vi "Rinocloud_explorer.vi"() -> ()   [LabVIEW 2013, in "Rinocloud Library.lvlib"]
uses:
  Rinocloud Library.lvlib
  Rinocloud_global_variable.vi
panel:
  out "Last action:":string
  out "error out":errorcluster
  in  "Active item:":string="<folder> home (id=)"
  in  "delete":bool
  in  "refresh list":bool
  in  "Tab Control":T1(tab)=enum."HTTP"
  in  "Cluster 2":T2={"Attribute"="", "Value"="", "Data type"=5} {"Data type" items=["Numeric", "String", "1D array of strings", "1D array of doubles", "Data JSON string", "<null>"]}
  in  "Cluster 1":T2={"Attribute"="", "Value"="", "Data type"=5} {"Data type" items=["Numeric", "String", "1D array of strings", "1D array of doubles", "Data JSON string", "<null>"]}
  in  "name":string
  in  "tags":string
  in  "notes":string
  in  "new folder":bool
  in  "upload file":bool
  in  "Name:":string
  in  "Tags:":string
  in  "Notes:":string
  in  "get metadata":bool
  in  "metadata tree":string(tree) caption="Metadata"
  in  "update metadata":bool
  in  "Move":bool
  in  "Destination:":string
  in  "Source:":string
  in  "set source":bool
  in  "set destination":bool
  out "body":string
  out "headers":string
  in  "ancestor tree":string(tree)="home" caption="Active path"
  in  "stop":bool
  in  "active child tree":string(tree) caption="File & folder list of the active folder"
  # "Double-click an item to activate"
  # "Custom metadata:"
  # "(tag1,tag2,tag3,...)"
  # "Click the fields to edit"
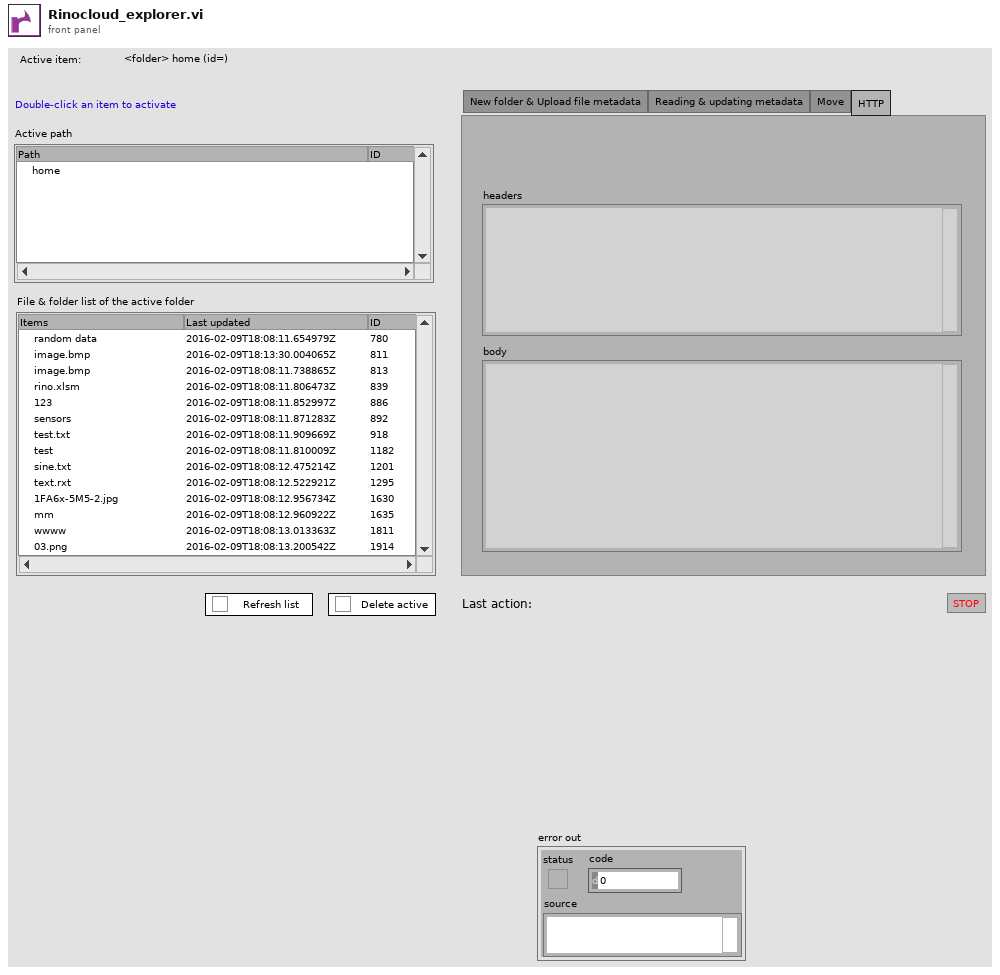
[diagram p1: front panel]
types:
  T1 = enum32{"New folder & Upload file metadata", "Reading & updating metadata", "Move", "HTTP"}
  T2 = cluster{"Attribute":string, "Value":string, "Data type":u16}
  T3 = cluster{"Active items":cluster{"Active file ID":string, "Active dir ID":string, "Active object ID":string, "Recent ID":string, "Active item:":string, "Source item":string, "Destination item":string, "Source ID":string, "Destination ID":string}, "Trees":cluster{"Ancestors":refnum<vi>, "Children":refnum<vi>, "Metadata":refnum<vi>}, "New metadata":cluster{"Name":string, "Tags":string, "Notes":string, "Custom metadata":cluster{"Attribute":string, "Value":string, "Data type":u16}[]}, "Communication":cluster{"HTTP headers":string, "HTTP body":string, "Project name":string, "User":string}, "Controls":cluster{"Move refnum":refnum<vi>}, "Status messages":cluster{"error ":errorcluster, "status":string}, "Update metadata":cluster{"Name":string, "Tags":string, "Notes":string}}
  T4 = enum16{"Boot", "Initialize", "Wait for event", "Refresh", "Metadata to tree", "Stop"}
  T5 = cluster{"Active file ID":string, "Active dir ID":string, "Active object ID":string, "Recent ID":string, "Active item:":string, "Source item":string, "Destination item":string, "Source ID":string, "Destination ID":string}
  T6 = enum8{"Enabled", "Disabled", "Disabled and Grayed Out"}
  T7 = cluster{"HTTP headers":string, "HTTP body":string, "Project name":string, "User":string}
  T8 = cluster{"Name":string, "Tags":string, "Notes":string, "Custom metadata":cluster{"Attribute":string, "Value":string, "Data type":u16}[]}
  T9 = enum16{"Boot", "Initialize", "Wait for event", "Refresh", "Stop"}
  T10 = cluster{"Store locally":bool, "ancestor array":cluster{"id":string, "name":string, "created_on":string, "updated_on":string, "tags":string, "notes":string, "record type":string, "metadata (JSON)":string}[], "Store metadata":bool}
  T11 = cluster{"Attribute":string, "Value":string, "Data type":enum16{"Numeric", "String", "1D array of strings", "1D array of doubles", "Data JSON string", "<null>"}}[]
  T12 = cluster{"headers":string, "body":string, "ID":string, "Saved":bool}
  T13 = cluster{"Attribute":string, "Value":string, "Data type":u16}[]
  T14 = cluster{"id":string, "name":string, "created_on":string, "updated_on":string, "tags":string, "notes":string, "record type":string, "metadata (JSON)":string}[]
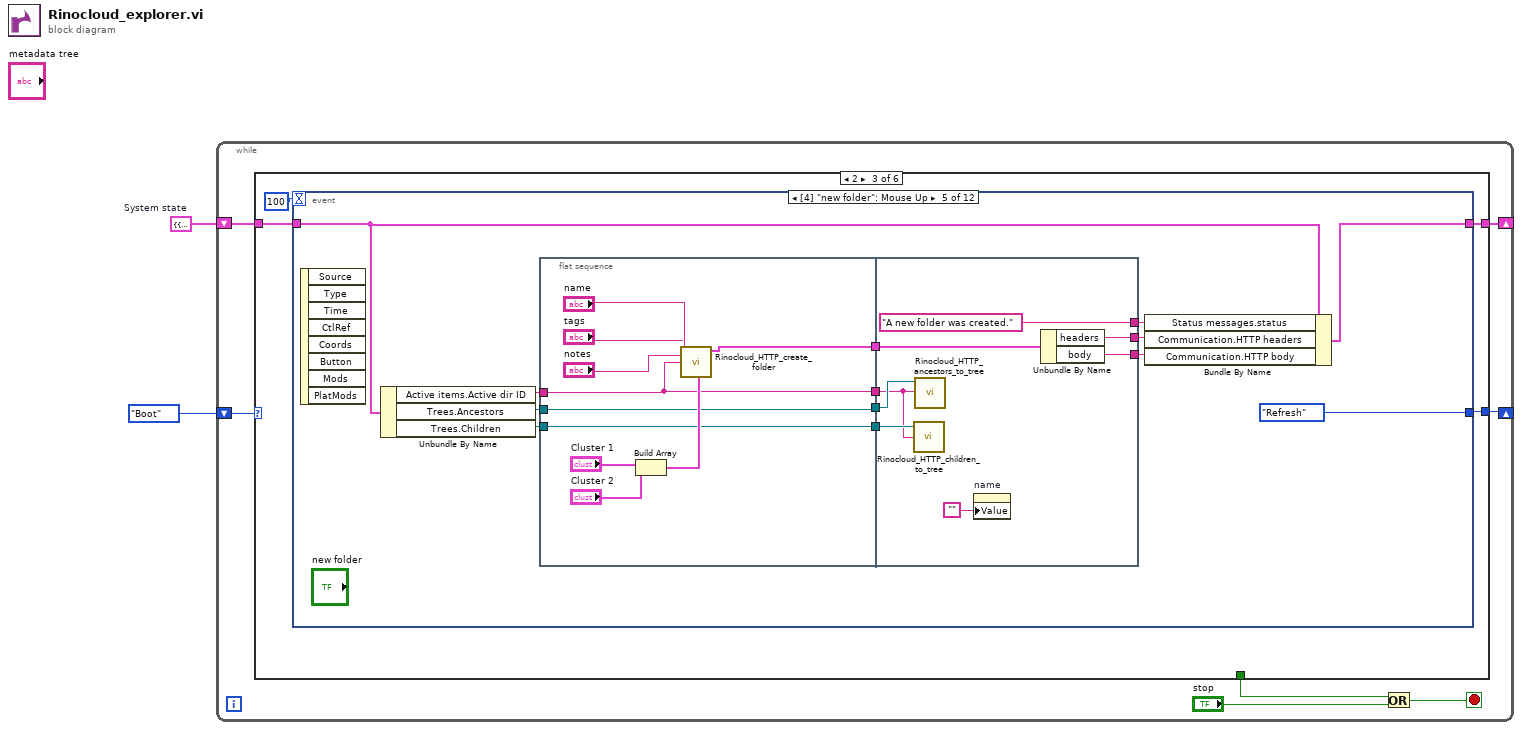
[diagram p0: block diagram]
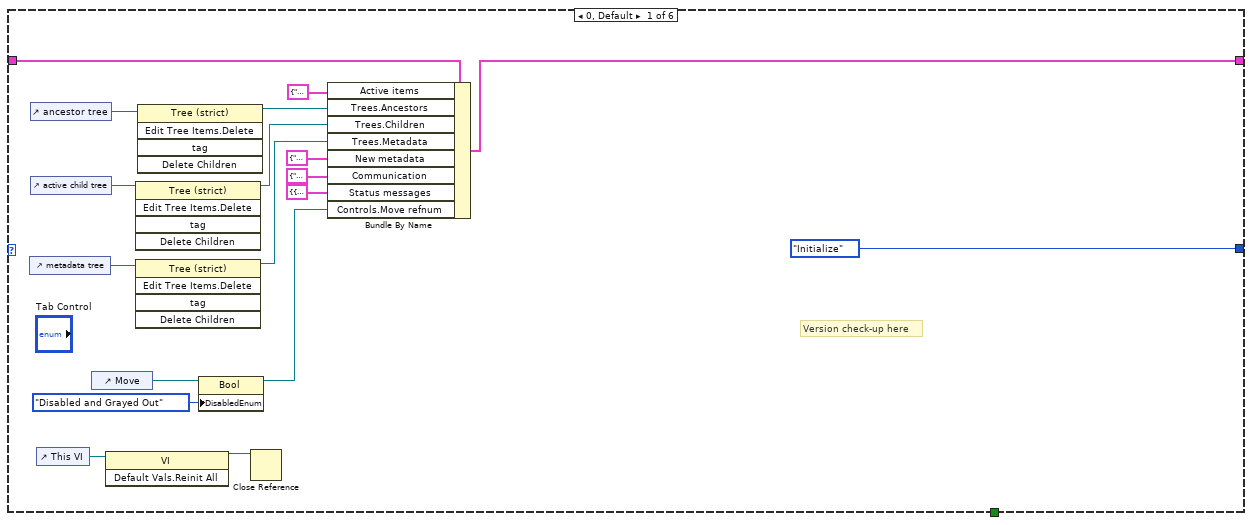
[diagram p2: hidden frame]
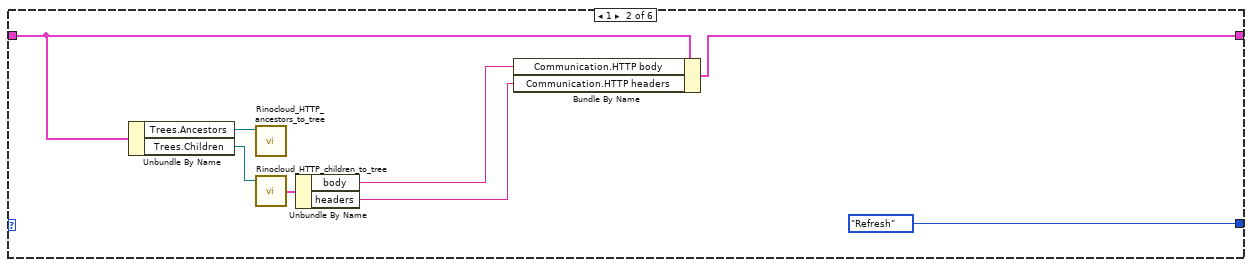
[diagram p3: hidden frame]
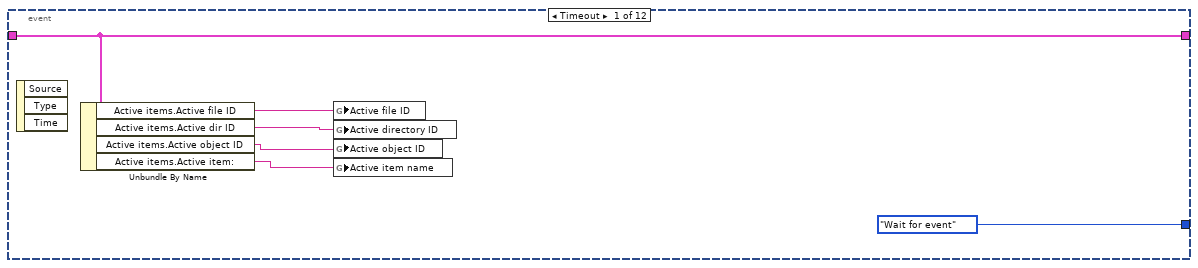
[diagram p4: hidden frame]
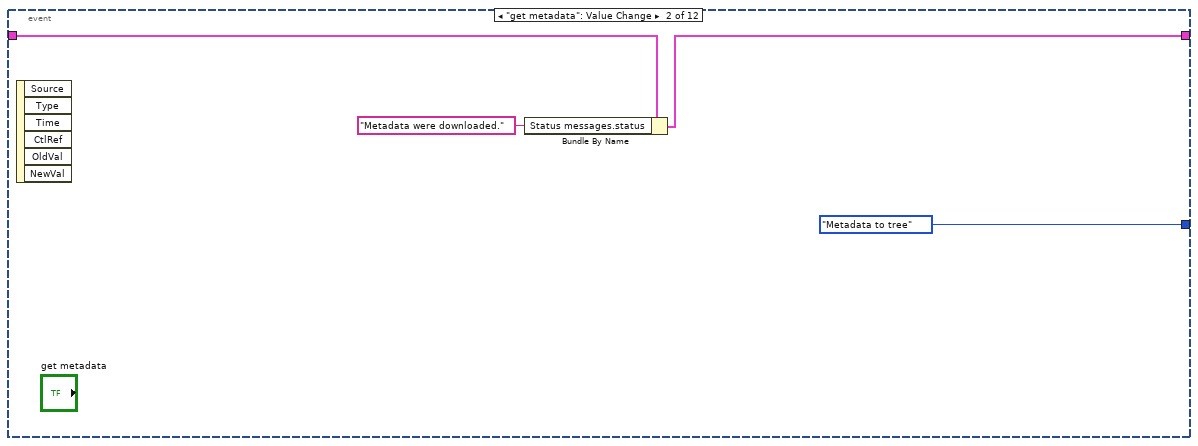
[diagram p5: hidden frame]
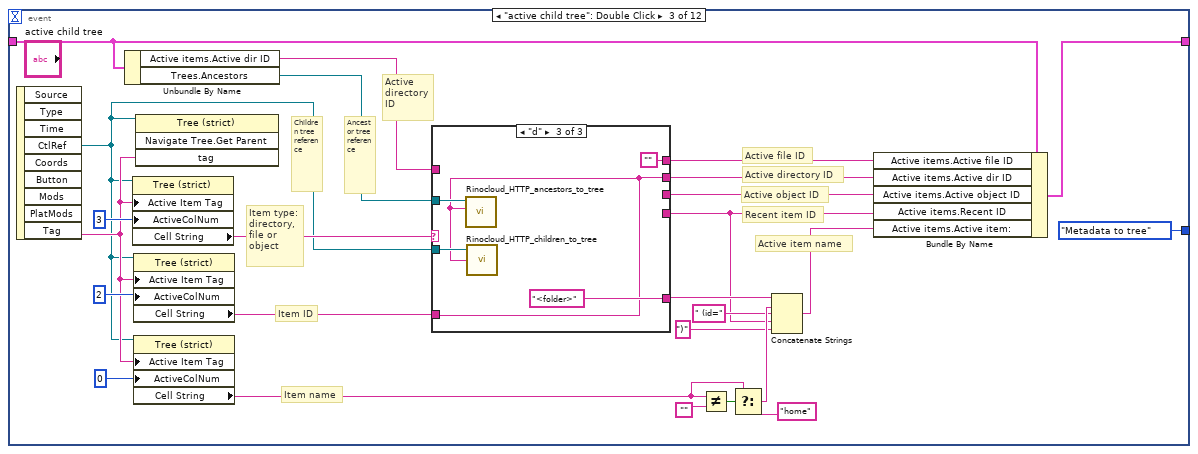
[diagram p6: hidden frame]
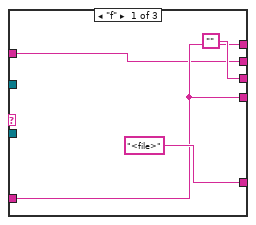
[diagram p7: hidden frame]
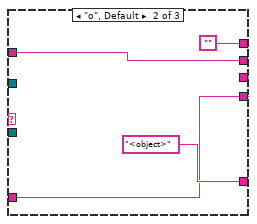
[diagram p8: hidden frame]
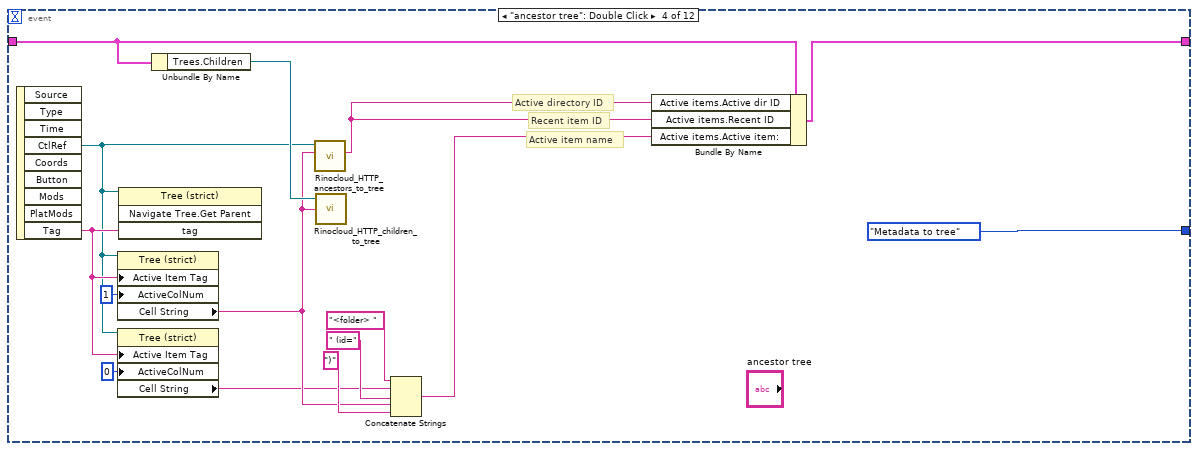
[diagram p9: hidden frame]
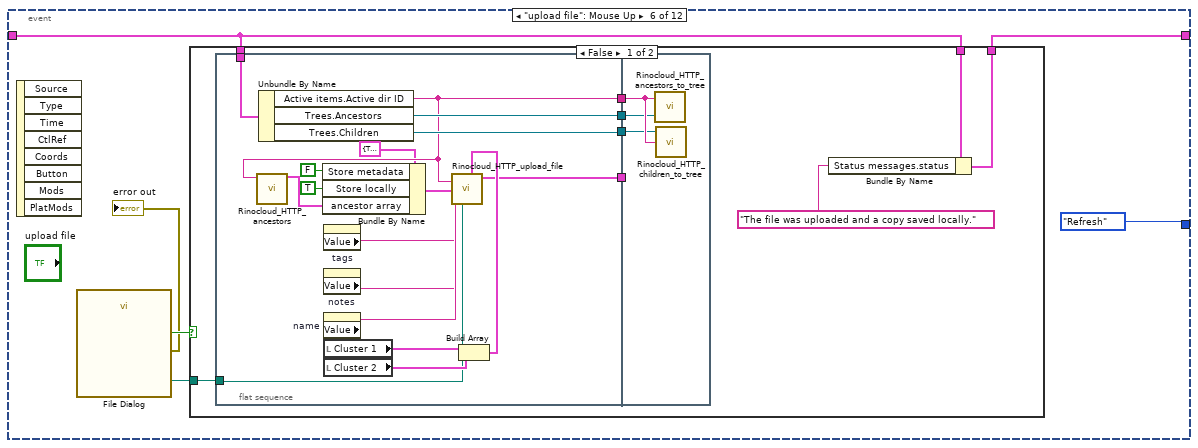
[diagram p10: hidden frame]
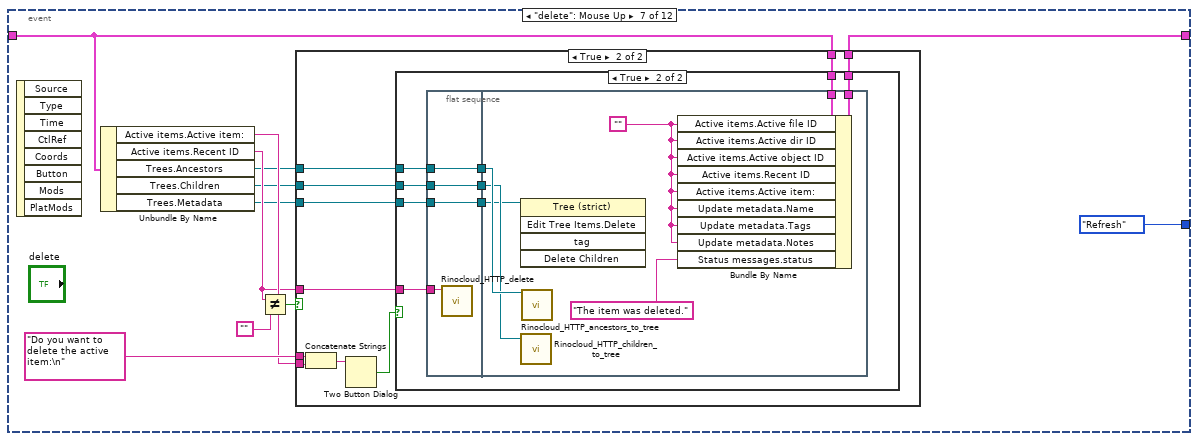
[diagram p12: hidden frame]
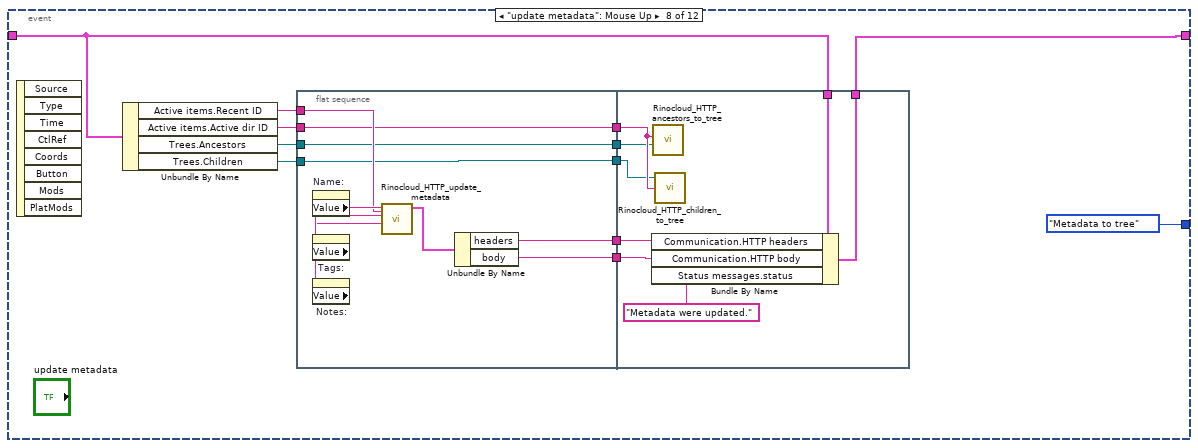
[diagram p15: hidden frame]
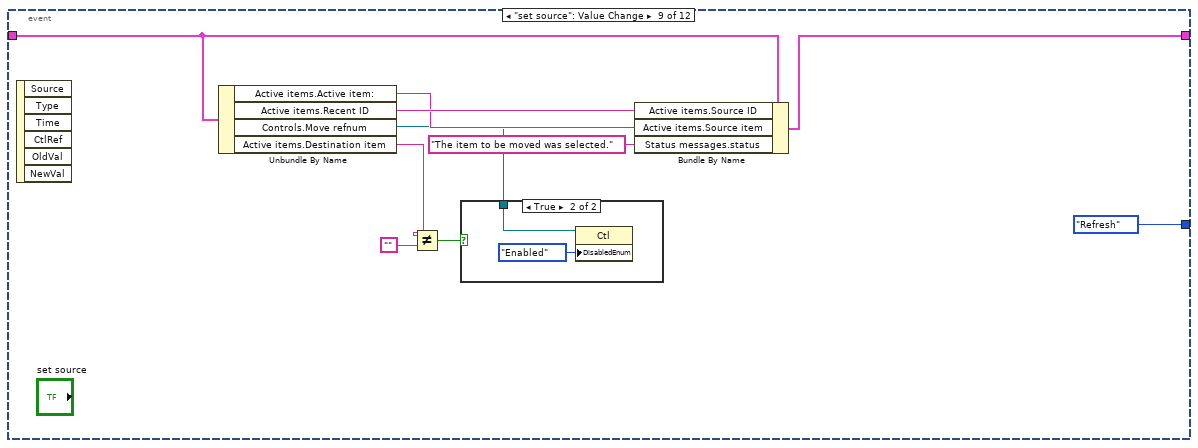
[diagram p16: hidden frame]
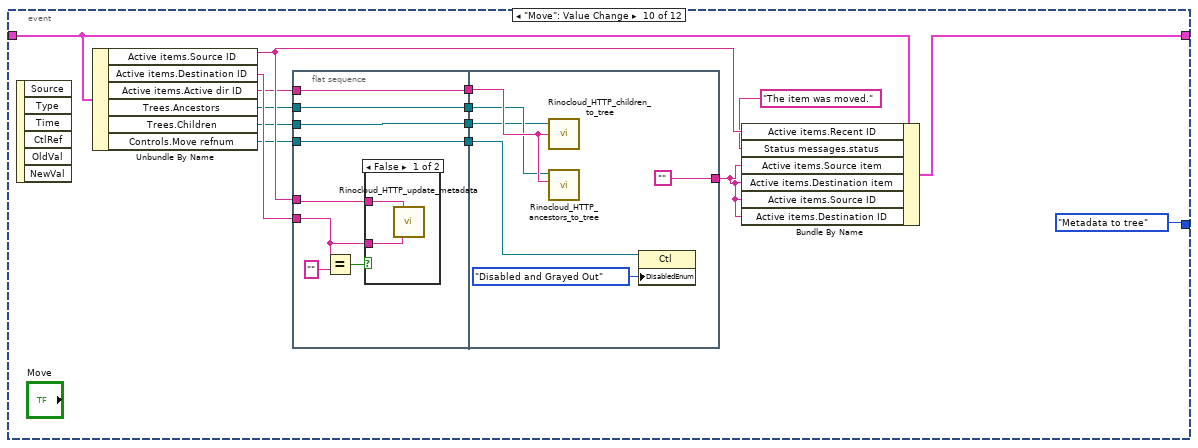
[diagram p18: hidden frame]
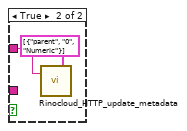
[diagram p19: hidden frame]
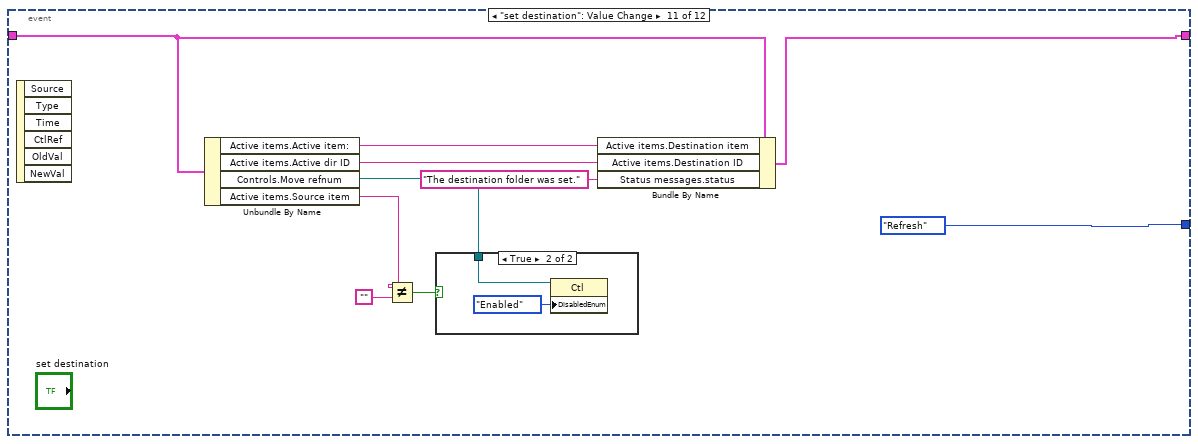
[diagram p20: hidden frame]
diagram:
  w2 = T3 {"Active items"={"Active file ID"="", "Active dir ID"="", "Active object ID"="", "Recent ID"="", "Active item:"="<folder> home (id=)", "Source item"="", "Destination item"="", "Source ID"="", "Destination ID"=""}, "Trees"={"Ancestors"=refnum, "Children"=refnum, "Metadata"=refnum}, "New metadata"={"Name"="", "Tags"="", "Notes"="", "Custom metadata"=[]}, "Communication"={"HTTP headers"="", "HTTP body"="", "Project name"="", "User"=""}, "Controls"={"Move refnum"=refnum}, "Status messages"={"error "={"status"=FALSE, "code"=0, "source"=""}, "status"=""}, "Update metadata"={"Name"="", "Tags"="", "Notes"=""}}  # System state
  n1 = while {
    shift-right: [w3] -> _
    shift-left: T4."Boot" -> [w9]
    shift-right: [w4] -> _
    shift-left: w2 -> [w5]
    stop <- w8 stop-if-true
    n2 = case shown="2" w9 {
      tunnel: [T4."Initialize" T9."Refresh" w38 T9."Wait for event" T4."Stop" T4."Refresh"] -> w3
      tunnel: [_ _ _ _ TRUE _] -> w6
      tunnel: w5 -> [w27 w32 w37 w312 w316 w324]
      tunnel: [w18 w29 w36 w312 w316 w323] -> w4
      frame 0, Default {
        # "Version check-up here"
        n3 = control-ref of="metadata tree"() -> (w22:refnum<vi>)
        n4 = control-ref of="ancestor tree"() -> (w26:refnum<vi>)
        n5 = control-ref of="active child tree"() -> (w24:refnum<vi>)
        n6 = control-ref of="This VI"() -> (w13:refnum<vi>)
        n7 = control-ref of="Move"() -> (w17:refnum<vi>)
        n8 = invoke class="VI" method="Default Vals.Reinit All"(reference=w13) -> (reference out=w12:refnum<vi>)  [unwired: 2 in, 2 out]
        n9 = invoke class="Tree (strict)" method="Edit Tree Items.Delete"(reference=w24) -> (reference out=w23:refnum<vi>)  [unwired: 4 in, 4 out]
        n10 = invoke class="Tree (strict)" method="Edit Tree Items.Delete"(reference=w22) -> (reference out=w11:refnum<vi>)  [unwired: 4 in, 4 out]
        n11 = invoke class="Tree (strict)" method="Edit Tree Items.Delete"(reference=w26) -> (reference out=w25:refnum<vi>)  [unwired: 4 in, 4 out]
        n12 = property class="Bool"(reference=w17, "DisabledEnum"=T6."Disabled and Grayed Out" ("Disabled")) -> (reference out=w15:refnum<vi>)  [unwired: 1 in, 1 out]
        n13 = Close Reference(reference=w12) -> ()  [unwired: 1 in, 1 out]
        n14 = Bundle By Name(cluster=w27, "Active items"=T5 {"Active file ID"="", "Active dir ID"="", "Active object ID"="", "Recent ID"="", "Active item:"="<folder> home (id=)", "Source item"="", "Destination item"="", "Source ID"="", "Destination ID"=""}, "Trees.Ancestors"=w25, "Trees.Children"=w23, "Trees.Metadata"=w11, "New metadata"=T8 {"Name"="", "Tags"="", "Notes"="", "Custom metadata"=[]} ("Metadata"), "Communication"=T7 {"HTTP headers"="", "HTTP body"="", "Project name"="", "User"=""}, "Status messages"=cluster{"error ":errorcluster, "status":string} {"error "={"status"=FALSE, "code"=0, "source"=""}, "status"=""}, "Controls.Move refnum"=w15) -> (w18:T3)
      }
      frame 1 {
        n15 = Unbundle By Name(w32) -> ("Trees.Ancestors"=w33:refnum<vi>, "Trees.Children"=w34:refnum<vi>)
        n16 = call "Rinocloud_HTTP_ancestors_to_tree.vi"("Tree Ref in"=w33) -> ()  [unwired: 3 in, 4 out]
        n17 = call "Rinocloud_HTTP_children_to_tree.vi"("Tree Ref in"=w34) -> ("Status"=w35:T12)  [unwired: 2 in, 2 out]
        n18 = Unbundle By Name(w35) -> ("body"=w31:string, "headers"=w30:string)
        n19 = Bundle By Name(cluster=w32, "Communication.HTTP body"=w31, "Communication.HTTP headers"=w30) -> (w29:T3)
      }
      frame 2 {
        n20 = event shown="[4] \"new folder\": Mouse Up" {
          selector: _ -> [_ _ _ _ _ _ _ _ _ _ _ _]
          dyn-events: _ -> [_ _ _ _ _ _ _ _ _ _ _ _]
          timeout: 100 -> [_ _ _ _ _ _ _ _ _ _ _ _]
          tunnel: [T9."Wait for event" T4."Metadata to tree" T4."Metadata to tree" T4."Metadata to tree" T4."Refresh" T4."Refresh" T4."Refresh" T4."Metadata to tree" T4."Refresh" T4."Metadata to tree" T4."Refresh" T4."Initialize"] -> w38
          tunnel: w37 -> [w40 w47 w62 w97 w108 w136 w172 w216 w252 w267 w292 w301]
          tunnel: [w40 w46 w59 w95 w107 w135 w170 w213 w244 w258 w288 w300] -> w36
          event Timeout {
            n21 = event-data() -> ()  [unwired: 1 in, 3 out]
            n22 = Unbundle By Name(w40) -> ("Active items.Active file ID"=w45:string, "Active items.Active dir ID"=w44:string, "Active items.Active object ID"=w43:string, "Active items.Active item:"=w41:string)
            n23 = global write "Rinocloud_global_variable.vi" "Active file ID"(w45) -> ()
            n24 = global write "Rinocloud_global_variable.vi" "Active directory ID"(w44) -> ()
            n25 = global write "Rinocloud_global_variable.vi" "Active object ID"(w43) -> ()
            n26 = global write "Rinocloud_global_variable.vi" "Active item name"(w41) -> ()
          }
          event "get metadata": Value Change {
            n27 = event-data() -> ()  [unwired: 1 in, 6 out]
            n28 = Bundle By Name(cluster=w47, "Status messages.status"="Metadata were downloaded.") -> (w46:T3)
          }
          event "active child tree": Double Click {
            # "Active \ndirectory\nID"
            # "Ancestor tree \nreference"
            # "Children tree \nreference"
            # "Item name"
            # "Item type:\ndirectory,\nfile or\nobject"
            # "Item ID"
            # "Active item name"
            # "Recent item ID"
            # "Active object ID"
            # "Active directory ID"
            # "Active file ID"
            n29 = event-data() -> ("CtlRef"=w50:refnum<vi>, "Tag"=w55:string)  [unwired: 1 in, 7 out]
            n30 = Unbundle By Name(w62) -> ("Active items.Active dir ID"=w60:string, "Trees.Ancestors"=w61:refnum<vi>)
            n31 = property on="Property Node" class="Tree (strict)"(reference=w50, "Active Item Tag"=w55, "ActiveColNum"=3 ("Active Cell:Active Column Number")) -> ("Cell String"=w54:string)  [unwired: 1 in, 2 out]
            n32 = property on="Property Node" class="Tree (strict)"(reference=w50, "Active Item Tag"=w55, "ActiveColNum"=2 ("Active Cell:Active Column Number")) -> ("Cell String"=w53:string)  [unwired: 1 in, 2 out]
            n33 = property on="Property Node" class="Tree (strict)"(reference=w50, "Active Item Tag"=w55, "ActiveColNum"=0 ("Active Cell:Active Column Number")) -> ("Cell String"=w52:string)  [unwired: 1 in, 2 out]
            n34 = invoke on="Invoke Node" class="Tree (strict)" method="Navigate Tree.Get Parent"(reference=w50, "tag"=w55) -> ()  [unwired: 2 in, 4 out]
            n35 = case shown="\"d\"" w54 {
              tunnel: w53 -> [w76 w81 w83]
              tunnel: ["<file>" ("f") "<object>" ("f") "<folder>" ("f")] -> w70
              tunnel: [w76 w81 w83] -> w64
              tunnel: ["" w81 w86] -> w65
              tunnel: [w76 "" w86] -> w51
              tunnel: [w75 w79 w83] -> w63
              tunnel: w61 -> [_ _ w85]
              tunnel: w50 -> [_ _ w84]
              tunnel: w60 -> [w75 w79 _]
              frame "f" {
              }
              frame "o", Default {
              }
              frame "d" {
                w86 = ""
                n36 = call "Rinocloud_HTTP_ancestors_to_tree.vi"("id"=w83, "Tree Ref in"=w85) -> ()  [unwired: 2 in, 4 out]
                n37 = call "Rinocloud_HTTP_children_to_tree.vi"("id"=w83, "Tree Ref in"=w84) -> ()  [unwired: 1 in, 3 out]
              }
            }
            n38 = Not Equal?(x=w52, y="") -> (x != y?=w72:bool)
            n39 = Select(t=w52, s=w72, f="home") -> (s? t:f=w69:string)
            n40 = Concatenate Strings(w70, w69, " (id=" ("string"), w64, ")" ("string")) -> (w66:string)
            n41 = Bundle By Name(cluster=w62, "Active items.Active file ID"=w51, "Active items.Active dir ID"=w63, "Active items.Active object ID"=w65, "Active items.Recent ID"=w64, "Active items.Active item:"=w66) -> (w59:T3)
          }
          event "ancestor tree": Double Click {
            # "Active item name"
            # "Recent item ID"
            # "Active directory ID"
            n42 = event-data() -> ("CtlRef"=w88:refnum<vi>, "Tag"=w91:string)  [unwired: 1 in, 7 out]
            n43 = property on="Property Node" class="Tree (strict)"(reference=w88, "Active Item Tag"=w91, "ActiveColNum"=1 ("Active Cell:Active Column Number")) -> ("Cell String"=w90:string)  [unwired: 1 in, 2 out]
            n44 = property on="Property Node" class="Tree (strict)"(reference=w88, "Active Item Tag"=w91, "ActiveColNum"=0 ("Active Cell:Active Column Number")) -> ("Cell String"=w89:string)  [unwired: 1 in, 2 out]
            n45 = invoke on="Invoke Node" class="Tree (strict)" method="Navigate Tree.Get Parent"(reference=w88, "tag"=w91) -> ()  [unwired: 2 in, 4 out]
            n46 = Unbundle By Name(w97) -> ("Trees.Children"=w98:refnum<vi>)
            n47 = call "Rinocloud_HTTP_ancestors_to_tree.vi"("id"=w90, "Tree Ref in"=w88) -> ("last ID"=w96:string)  [unwired: 2 in, 3 out]
            n48 = call "Rinocloud_HTTP_children_to_tree.vi"("id"=w90, "Tree Ref in"=w98) -> ()  [unwired: 1 in, 3 out]
            n49 = Concatenate Strings("<folder> " ("string"), w89, " (id=" ("string"), w90, ")" ("string")) -> (w94:string)
            n50 = Bundle By Name(cluster=w97, "Active items.Active dir ID"=w96, "Active items.Recent ID"=w96, "Active items.Active item:"=w94) -> (w95:T3)
          }
          event "new folder": Mouse Up {
            n51 = event-data() -> ()  [unwired: 1 in, 8 out]
            n52 = Unbundle By Name(w108) -> ("Active items.Active dir ID"=w114:string, "Trees.Ancestors"=w113:refnum<vi>, "Trees.Children"=w112:refnum<vi>)
            n53 = flat-sequence {
              tunnel: w114 -> [w124]
              tunnel: w113 -> [w123]
              tunnel: w112 -> [w122]
              tunnel: [w124] -> w111
              tunnel: [w123] -> w110
              tunnel: [w122] -> w109
              tunnel: [w121] -> w106
              tunnel: w111 -> [w130]
              tunnel: w110 -> [w132]
              tunnel: w109 -> [w131]
              tunnel: w106 -> [w129]
              tunnel: [w128] -> w105
              tunnel: [w127] -> w104
              tunnel: ["A new folder was created." ("Status messages.status")] -> w103
              frame #0 {
                n54 = Build Array("Cluster 1", "Cluster 2") -> (w125:T13)
                n55 = call "Rinocloud_HTTP_create_folder.vi"("Extra metadata array"=w125, "Parent ID"=w124, "Notes"="notes", "Tags"="tags", "Name"="name") -> ("Status"=w121:T12)  [unwired: 3 in, 1 out]
              }
              frame #1 {
                n56 = call "Rinocloud_HTTP_children_to_tree.vi"("id"=w130, "Tree Ref in"=w131) -> ()  [unwired: 1 in, 3 out]
                n57 = call "Rinocloud_HTTP_ancestors_to_tree.vi"("id"=w130, "Tree Ref in"=w132) -> ()  [unwired: 2 in, 4 out]
                n58 = property on="name" class="Str"("Value"="") -> ()  [unwired: 2 in, 2 out]
                n59 = Unbundle By Name(w129) -> ("headers"=w128:string, "body"=w127:string)
              }
            }
            n60 = Bundle By Name(cluster=w108, "Status messages.status"=w103, "Communication.HTTP headers"=w105, "Communication.HTTP body"=w104) -> (w107:T3)
          }
          event "upload file": Mouse Up {
            n61 = event-data() -> ()  [unwired: 1 in, 8 out]
            n62 = call "File Dialog"() -> ("selected path"=w138:path, "cancelled"=w139:bool, "error out"=→"error out":errorcluster)  [unwired: 12 in, 1 out]
            n63 = case shown="False" w139 {
              tunnel: w138 -> [w148 _]
              tunnel: w136 -> [w147 _]
              tunnel: w136 -> [w142 w169]
              tunnel: [w140 w169] -> w135
              frame False {
                n64 = flat-sequence {
                  tunnel: w148 -> [w163]
                  tunnel: w147 -> [w156]
                  tunnel: [w155] -> w146
                  tunnel: [w154] -> w145
                  tunnel: [w153] -> w144
                  tunnel: [w152] -> w143
                  tunnel: w146 -> [w166]
                  tunnel: w145 -> [w167]
                  tunnel: w144 -> [_]
                  tunnel: w143 -> [w168]
                  frame #0 {
                    n65 = Unbundle By Name(w156) -> ("Active items.Active dir ID"=w152:string, "Trees.Ancestors"=w155:refnum<vi>, "Trees.Children"=w154:refnum<vi>)
                    n66 = call "Rinocloud_HTTP_ancestors.vi"("id"=w152) -> ("metadata array"=w157:T14)  [unwired: 3 in, 3 out]
                    n67 = Bundle By Name(cluster=T10 {"Store locally"=TRUE, "ancestor array"=[], "Store metadata"=TRUE} ("local storage"), "Store metadata"=FALSE ("Store locally"), "Store locally"=TRUE, "ancestor array"=w157) -> (w149:T10)
                    n68 = property on="tags" class="Str"() -> ("Value"=w161:string)  [unwired: 2 in, 2 out]
                    n69 = property on="notes" class="Str"() -> ("Value"=w160:string)  [unwired: 2 in, 2 out]
                    n70 = property on="name" class="Str"() -> ("Value"=w162:string)  [unwired: 2 in, 2 out]
                    n71 = local read "Cluster 1"() -> (w165:T2)
                    n72 = local read "Cluster 2"() -> (w164:T2)
                    n73 = Build Array(w165, w164) -> (w159:T13)
                    n74 = call "Rinocloud_HTTP_upload_file.vi"("local storage"=w149, "Extra metadata array"=w159, "Path in"=w163, "Parent ID"=w152, "Notes"=w160, "Tags"=w161, "Name"=w162) -> ("Status"=w153:T12)  [unwired: 2 in, 2 out]
                  }
                  frame #1 {
                    n75 = call "Rinocloud_HTTP_ancestors_to_tree.vi"("id"=w168, "Tree Ref in"=w166) -> ()  [unwired: 2 in, 4 out]
                    n76 = call "Rinocloud_HTTP_children_to_tree.vi"("id"=w168, "Tree Ref in"=w167) -> ()  [unwired: 1 in, 3 out]
                  }
                }
                n77 = Bundle By Name(cluster=w142, "Status messages.status"="The file was uploaded and a copy saved locally.") -> (w140:T3)
              }
              frame True {
              }
            }
          }
          event "delete": Mouse Up {
            n78 = event-data() -> ()  [unwired: 1 in, 8 out]
            n79 = Unbundle By Name(w172) -> ("Active items.Active item:"=w177:string, "Active items.Recent ID"=w176:string, "Trees.Ancestors"=w175:refnum<vi>, "Trees.Children"=w174:refnum<vi>, "Trees.Metadata"=w173:refnum<vi>)
            n80 = Not Equal?(x=w176, y="") -> (x != y?=w180:bool)
            n81 = case shown="True" w180 {
              tunnel: w176 -> [_ w189]
              tunnel: "Do you want to delete the active item:\n" ("message") -> [_ w188]
              tunnel: w177 -> [_ w187]
              tunnel: w175 -> [_ w186]
              tunnel: w174 -> [_ w185]
              tunnel: w173 -> [_ w184]
              tunnel: w172 -> [w181 w183]
              tunnel: [w181 w182] -> w170
              frame False {
              }
              frame True {
                n82 = Concatenate Strings(w188, w187) -> (w191:string)
                n83 = Two Button Dialog(message=w191) -> (T button?=w190:bool)  [unwired: 2 in]
                n84 = case shown="True" w190 {
                  tunnel: w189 -> [_ w201]
                  tunnel: w186 -> [_ w199]
                  tunnel: w185 -> [_ w197]
                  tunnel: w184 -> [_ w195]
                  tunnel: w183 -> [w192 w194]
                  tunnel: [w192 w193] -> w182
                  frame False {
                  }
                  frame True {
                    n85 = flat-sequence {
                      tunnel: w201 -> [w205]
                      tunnel: [w204] -> w200
                      tunnel: w199 -> [w204]
                      tunnel: [w203] -> w198
                      tunnel: w197 -> [w203]
                      tunnel: [w202] -> w196
                      tunnel: w195 -> [w202]
                      tunnel: w200 -> [w212]
                      tunnel: w198 -> [w211]
                      tunnel: w196 -> [w210]
                      tunnel: w194 -> [w209]
                      tunnel: [w206] -> w193
                      frame #0 {
                        n86 = call "Rinocloud_HTTP_delete.vi"("ID"=w205) -> ()  [unwired: 6 in, 2 out]
                      }
                      frame #1 {
                        w208 = ""
                        n87 = invoke class="Tree (strict)" method="Edit Tree Items.Delete"(reference=w210) -> ()  [unwired: 4 in, 5 out]
                        n88 = call "Rinocloud_HTTP_children_to_tree.vi"("Tree Ref in"=w211) -> ()  [unwired: 2 in, 3 out]
                        n89 = call "Rinocloud_HTTP_ancestors_to_tree.vi"("Tree Ref in"=w212) -> ()  [unwired: 3 in, 4 out]
                        n90 = Bundle By Name(cluster=w209, "Active items.Active file ID"=w208, "Active items.Active dir ID"=w208, "Active items.Active object ID"=w208, "Active items.Recent ID"=w208, "Active items.Active item:"=w208, "Update metadata.Name"=w208, "Update metadata.Tags"=w208, "Update metadata.Notes"=w208, "Status messages.status"="The item was deleted.") -> (w206:T3)
                      }
                    }
                  }
                }
              }
            }
          }
          event "update metadata": Mouse Up {
            n91 = event-data() -> ()  [unwired: 1 in, 8 out]
            n92 = Unbundle By Name(w216) -> ("Active items.Recent ID"=w224:string, "Active items.Active dir ID"=w222:string, "Trees.Ancestors"=w220:refnum<vi>, "Trees.Children"=w217:refnum<vi>)
            n93 = flat-sequence {
              tunnel: w224 -> [w231]
              tunnel: [w230] -> w223
              tunnel: w222 -> [w230]
              tunnel: w220 -> [w229]
              tunnel: [w229] -> w219
              tunnel: [w228] -> w218
              tunnel: w217 -> [w228]
              tunnel: [w226] -> w215
              tunnel: [w225] -> w214
              tunnel: w223 -> [w242]
              tunnel: w219 -> [w240]
              tunnel: w218 -> [w241]
              tunnel: w216 -> [w239]
              tunnel: w215 -> [w237]
              tunnel: w214 -> [w236]
              tunnel: [w235] -> w213
              frame #0 {
                n94 = property on="Name:" class="Str"() -> ("Value"=w232:string)  [unwired: 2 in, 2 out]
                n95 = property on="Tags:" class="Str"() -> ("Value"=w234:string)  [unwired: 2 in, 2 out]
                n96 = property on="Notes:" class="Str"() -> ("Value"=w233:string)  [unwired: 2 in, 2 out]
                n97 = call "Rinocloud_HTTP_update_metadata.vi"("self ID"=w231, "Notes"=w233, "Tags"=w234, "Name"=w232) -> ("Status"=w227:T12)  [unwired: 6 in, 1 out]
                n98 = Unbundle By Name(w227) -> ("headers"=w226:string, "body"=w225:string)
              }
              frame #1 {
                n99 = Bundle By Name(cluster=w239, "Communication.HTTP headers"=w237, "Communication.HTTP body"=w236, "Status messages.status"="Metadata were updated.") -> (w235:T3)
                n100 = call "Rinocloud_HTTP_ancestors_to_tree.vi"("id"=w242, "Tree Ref in"=w240) -> ()  [unwired: 2 in, 4 out]
                n101 = call "Rinocloud_HTTP_children_to_tree.vi"("id"=w242, "Tree Ref in"=w241) -> ()  [unwired: 1 in, 3 out]
              }
            }
          }
          event "set source": Value Change {
            n102 = event-data() -> ()  [unwired: 1 in, 6 out]
            n103 = Unbundle By Name(w252) -> ("Active items.Active item:"=w250:string, "Active items.Recent ID"=w251:string, "Controls.Move refnum"=w247:refnum<vi>, "Active items.Destination item"=w248:string)
            n104 = Not Equal?(x=w248, y="") -> (x != y?=w246:bool)
            n105 = case shown="True" w246 {
              tunnel: w247 -> [_ w253]
              frame False {
              }
              frame True {
                n106 = property class="Ctl"(reference=w253, "DisabledEnum"=T6."Enabled" ("Disabled")) -> ()  [unwired: 1 in, 2 out]
              }
            }
            n107 = Bundle By Name(cluster=w252, "Active items.Source ID"=w251, "Active items.Source item"=w250, "Status messages.status"="The item to be moved was selected.") -> (w244:T3)
          }
          event "Move": Value Change {
            n108 = event-data() -> ()  [unwired: 1 in, 6 out]
            n109 = Unbundle By Name(w267) -> ("Active items.Source ID"=w266:string, "Active items.Destination ID"=w268:string, "Active items.Active dir ID"=w264:string, "Trees.Ancestors"=w262:refnum<vi>, "Trees.Children"=w260:refnum<vi>, "Controls.Move refnum"=w256:refnum<vi>)
            n110 = flat-sequence {
              tunnel: w266 -> [w275]
              tunnel: w268 -> [w274]
              tunnel: [w273] -> w265
              tunnel: w264 -> [w273]
              tunnel: [w272] -> w263
              tunnel: w262 -> [w272]
              tunnel: [w271] -> w261
              tunnel: w260 -> [w271]
              tunnel: [w270] -> w257
              tunnel: w256 -> [w270]
              tunnel: w265 -> [w287]
              tunnel: w263 -> [w286]
              tunnel: w261 -> [w285]
              tunnel: w257 -> [w284]
              tunnel: [""] -> w255
              frame #0 {
                n111 = Equal?(x=w274, y="") -> (x = y?=w276:bool)
                n112 = case shown="False" w276 {
                  tunnel: w275 -> [w279 w281]
                  tunnel: w274 -> [w278 _]
                  frame False {
                    n113 = call "Rinocloud_HTTP_update_metadata.vi"("parent ID"=w278, "self ID"=w279) -> ()  [unwired: 8 in, 2 out]
                  }
                  frame True {
                    n114 = call "Rinocloud_HTTP_update_metadata.vi"("Extra metadata array"=T11 [{"Attribute"="parent", "Value"="0", "Data type"=enum."Numeric"}], "self ID"=w281) -> ()  [unwired: 8 in, 2 out]
                  }
                }
              }
              frame #1 {
                n115 = call "Rinocloud_HTTP_children_to_tree.vi"("id"=w287, "Tree Ref in"=w285) -> ()  [unwired: 1 in, 3 out]
                n116 = call "Rinocloud_HTTP_ancestors_to_tree.vi"("id"=w287, "Tree Ref in"=w286) -> ()  [unwired: 2 in, 4 out]
                n117 = property class="Ctl"(reference=w284, "DisabledEnum"=T6."Disabled and Grayed Out" ("Disabled")) -> ()  [unwired: 1 in, 2 out]
              }
            }
            n118 = Bundle By Name(cluster=w267, "Active items.Recent ID"=w266, "Status messages.status"="The item was moved.", "Active items.Source item"=w255, "Active items.Destination item"=w255, "Active items.Source ID"=w255, "Active items.Destination ID"=w255) -> (w258:T3)
          }
          event "set destination": Value Change {
            n119 = event-data() -> ()  [unwired: 1 in, 6 out]
            n120 = Unbundle By Name(w292) -> ("Active items.Active item:"=w291:string, "Active items.Active dir ID"=w297:string, "Controls.Move refnum"=w294:refnum<vi>, "Active items.Source item"=w295:string)
            n121 = Not Equal?(x=w295, y="") -> (x != y?=w293:bool)
            n122 = case shown="True" w293 {
              tunnel: w294 -> [_ w298]
              frame False {
              }
              frame True {
                n123 = property class="Ctl"(reference=w298, "DisabledEnum"=T6."Enabled" ("Disabled")) -> ()  [unwired: 1 in, 2 out]
              }
            }
            n124 = Bundle By Name(cluster=w292, "Active items.Destination item"=w291, "Active items.Destination ID"=w297, "Status messages.status"="The destination folder was set.") -> (w288:T3)
          }
          event "refresh list": Mouse Up {
            n125 = event-data() -> ()  [unwired: 1 in, 8 out]
            n126 = Bundle By Name(cluster=w301, "Status messages.status"="The file list view was refreshed.") -> (w300:T3)
          }
        }
      }
      frame 3 {
        n127 = Unbundle By Name(w312) -> ("Update metadata.Name"=w306:string, "Update metadata.Tags"=w305:string, "Update metadata.Notes"=w304:string, "Communication.HTTP headers"=→"headers":string, "Communication.HTTP body"=→"body":string, "Status messages.status"=→"Last action:":string, "Active items.Active item:"=w309:string, "Active items.Source item"=w308:string, "Active items.Destination item"=w307:string)
        n128 = local write "Name:"(w306) -> ()
        n129 = local write "Tags:"(w305) -> ()
        n130 = local write "Notes:"(w304) -> ()
        n131 = local write "Active item:"(w309) -> ()
        n132 = local write "Source:"(w308) -> ()
        n133 = local write "Destination:"(w307) -> ()
      }
      frame 5 {
      }
      frame 4 {
        n134 = Unbundle By Name(w324) -> ("Active items.Recent ID"=w318:string, "Trees.Metadata"=w332:refnum<vi>)
        n135 = Not Equal?(x=w318, y="") -> (x != y?=w320:bool)
        n136 = Concatenate Strings("Metadata downloaded (id=" ("Communication.Project name"), w318, ")." ("string")) -> (w319:string)
        n137 = case shown="True" w320 {
          tunnel: w332 -> [w334 w342]
          tunnel: [w333 w341] -> w331
          tunnel: [w333 w340] -> w330
          tunnel: [w333 w339] -> w329
          tunnel: [w333 w338] -> w328
          tunnel: [w333 w337] -> w327
          tunnel: [w333 w336] -> _
          tunnel: w319 -> [_ w336]
          tunnel: w318 -> [_ w335]
          frame False {
            w333 = ""
            n138 = invoke class="Tree (strict)" method="Edit Tree Items.Delete"(reference=w334) -> ()  [unwired: 4 in, 5 out]
          }
          frame True {
            n139 = call "Rinocloud_HTTP_metadata_to_tree.vi"("JSON Tree Expanded Reference"=w342, "id"=w335) -> ("Notes"=w339:string, "Tags"=w340:string, "Name"=w341:string, "Status"=w343:T12)  [unwired: 4 in, 2 out]
            n140 = Unbundle By Name(w343) -> ("headers"=w338:string, "body"=w337:string)
          }
        }
        n141 = Bundle By Name(cluster=w324, "Update metadata.Name"=w331, "Update metadata.Tags"=w330, "Update metadata.Notes"=w329, "Communication.HTTP headers"=w328, "Communication.HTTP body"=w327) -> (w323:T3)
      }
    }
    n142 = Or(x=w6, y="stop") -> (x .or. y?=w8:bool)
  }
